vi "GenerateRandomNumber.vi"(8 "error in (no error)":errorcluster, 11 "RandomNumberModel in":refnum<class "RandomNumberModel.lvclass">) -> (0 "error out":errorcluster, 3 "RandomNumberModel out":refnum<class "RandomNumberModel.lvclass">)   [LabVIEW 2017, in "RandomNumberModel.lvlib" / "RandomNumberModel.lvclass"]
uses:
  <vilib>/gpm_packages/@cs/example/Dynamic Viewables/SequenceSteps/RandomNumberModel/RandomNumberModel.lvclass
  C:/Program Files/National Instruments/LabVIEW 2017/vi.lib/gpm_packages/@cs/mva-core/Source/IModel/IModel/IModel.lvclass
  C:/Program Files/National Instruments/LabVIEW 2017/vi.lib/ActorFramework/Actor/Actor.lvclass
  <vilib>/gpm_packages/@cs/mva-core/Source/IObserver/IObserver/IObserver.lvclass/IObserver.ctl
  <vilib>/gpm_packages/@cs/mva-core/Source/IModel/IModel/IModel.lvclass/IModel.ctl
  <vilib>/gpm_packages/@cs/mva-core/Source/IMediator/PublishRequest/PublishRequest.lvclass/PublishRequest.ctl
  <vilib>/gpm_packages/@cs/mva-core/Source/IMediator/IMediator Messages/Publish Msg/Publish Msg.lvclass/Publish Msg.ctl
  <vilib>/gpm_packages/@cs/actor-framework-messages/Source/RoundTripMessage/RoundTripMessage.lvclass/RoundTripMessage.ctl
  <vilib>/ActorFramework/Message Enqueuer/Message Enqueuer.lvclass/Message Enqueuer.ctl
  <vilib>/ActorFramework/Actor/Actor.lvclass/Actor.ctl
  <vilib>/gpm_packages/@cs/example/Dynamic Viewables/SequenceSteps/RandomNumberModel/RandomNumberModel.lvclass/RandomNumberModel.ctl
  cb7bf9b9-956b-4f49-b468-f64f0c203643.vi
  <vilib>/gpm_packages/@cs/mva-core/Source/IMediator/IMediator Messages/Publish Msg/Send Pre-Addressed Publish.vi
  <vilib>/gpm_packages/@cs/mva-core/Source/IObserver/IObserver/Read Unique ID.vi
  <vilib>/gpm_packages/@cs/mva-core/Source/IMediator/PublishRequest/Pack Publish Request.vi
  <vilib>/ActorFramework/Message Enqueuer/Init from Existing Queue.vi
  <vilib>/ActorFramework/Message Enqueuer/Enqueue.vi
  <vilib>/gpm_packages/@cs/actor-framework-messages/Source/RoundTripMessage/Return Round-Trip Message.vi
  <vilib>/gpm_packages/@cs/mva-core/Source/IModel/IModel/IModel.lvclass
  C:/Program Files/National Instruments/LabVIEW 2017/vi.lib/gpm_packages/@cs/mva-core/Source/IObserver/IObserver/IObserver.lvclass
  <vilib>/gpm_packages/@cs/mva-core/Source/IMediator/IMediator Messages/Publish Msg/Publish Msg.lvclass
  C:/Program Files/National Instruments/LabVIEW 2017/vi.lib/gpm_packages/@cs/actor-framework-messages/Source/RoundTripMessage/RoundTripMessage.lvclass
  <vilib>/gpm_packages/@cs/actor-framework-messages/Source/RoundTripMessage/RoundTripMessage.lvclass
  C:/Program Files/National Instruments/LabVIEW 2017/vi.lib/ActorFramework/Message/Message.lvclass
  <vilib>/ActorFramework/Stop Msg/Stop Msg.lvclass
  <vilib>/gpm_packages/@cs/example/Dynamic Viewables/SequenceSteps/RandomNumberModel Messages/GenerateRandomNumber Msg/GenerateRandomNumber Msg.lvclass
  <vilib>/Utility/error.llb/Error Cluster From Error Code.vi
  <vilib>/ActorFramework/Message Priority Queue/Priority Enqueue.vi
  <vilib>/gpm_packages/@cs/mva-core/Source/IMediator/PublishRequest/PublishRequest.lvclass
  <vilib>/ActorFramework/Message Enqueuer/Message Enqueuer.lvclass
  <vilib>/ActorFramework/Actor/Actor.lvclass
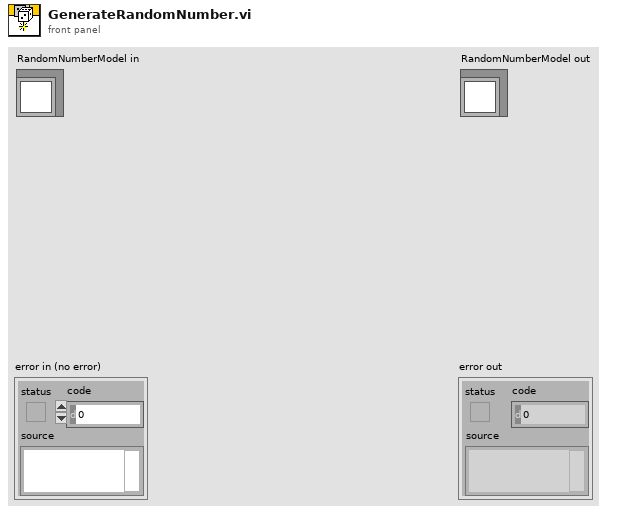
[diagram p1: front panel]
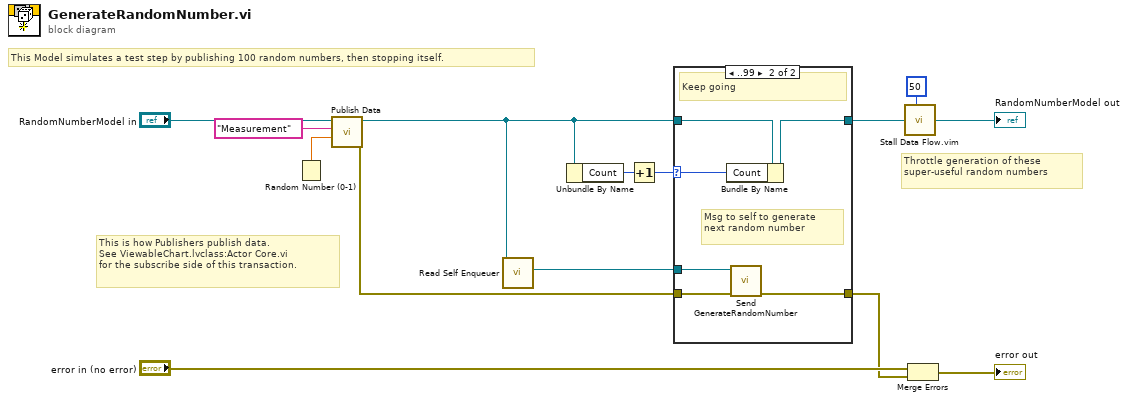
[diagram p0: block diagram]
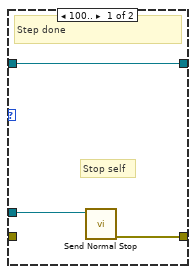
[diagram p2: hidden frame]
diagram:
  # "Throttle generation of these\nsuper-useful random numbers"
  # "This Model simulates a test step by publishing 100 random numbers, then stopping itself."
  # "This is how Publishers publish data.\nSee ViewableChart.lvclass:Actor Core.vi\nfor the subscribe side of this transaction."
  n1 = Random Number (0-1)() -> (number: 0 to 1=w11:dbl)
  n2 = call <vilib>:"Publish Data.vi"("Data to Publish"=w11, "Datum Name"="Measurement", "IModel in"="RandomNumberModel in") -> ("error out"=w9:errorcluster, "IModel out"=w4:refnum<class "RandomNumberModel.lvclass">)  [unwired: 7 in]
  n3 = call <vilib>:"Read Self Enqueuer.vi"("Actor"=w4) -> ("Self Enqueuer"=w8:refnum<class "Message Enqueuer.lvclass">)  [unwired: 10 in]
  n4 = Unbundle By Name(w4) -> ("Count"=w3:i32)
  n5 = Increment(x=w3) -> (x+1=w2:i32)
  n6 = case shown="..99" w2 {
    selector: w2 -> [_ w18]
    tunnel: w9 -> [_ w23]
    tunnel: w8 -> [w16 w22]
    tunnel: [w15 w21] -> w7
    tunnel: w4 -> [w17 w20]
    tunnel: [w17 w19] -> w1
    frame 100.. {
      # "Stop self"
      # "Step done"
      n7 = call <vilib>:"Send Normal Stop.vi"("Message Enqueuer"=w16) -> ("error out"=w15:errorcluster)  [unwired: 10 in]
    }
    frame ..99 {
      # "Msg to self to generate\nnext random number"
      # "Keep going"
      n8 = Bundle By Name(cluster=w20, "Count"=w18) -> (w19:refnum<class "RandomNumberModel.lvclass">)
      n9 = call <vilib>:"Send GenerateRandomNumber.vi"("error in (no error)"=w23, "Message Enqueuer"=w22) -> ("error out"=w21:errorcluster)  [unwired: 8 in, 1 out]
    }
  }
  n10 = call "Stall Data Flow.vim"("value in"=w1, "milliseconds to wait"=u32 50) -> ("value out"=→"RandomNumberModel out":refnum<class "RandomNumberModel.lvclass">)  [unwired: 1 out]
  n11 = Merge Errors("error in (no error)", w7) -> (→"error out":errorcluster)
